vi "ORS_AlazarDLLCfg_All.vi"(2 "Bad Clock Duration":dbl=2.05e-06, 3 "Good Clock Duration":dbl=2.65e-06, 4 "DESmode":bool, 6 "IgnoreBadClk":bool, 7 "ATS_clock":T1={"Source"=2, "Sample Rate"=48, "Edge"=0, "Rate Ext Ref"=400000000, "Trigger Delay"=0, "Rate Int Ref"=450} {"Rate Ext Ref" items=["0.4G"=400000000, "0.8G"=800000000, "1.2G"=1200000000, "1.6G"=1600000000, "2.0G"=2000000000, "2.4G"=2400000000, "2.8G"=2800000000, "3.2G"=3200000000, "3.6G"=3600000000]; "Edge" items=["Rising", "Falling"]; "Sample Rate" items=["1 kS/s"=1, "2 kS/s"=2, "5 kS/s"=4, "10 kS/s"=8, "20 kS/s"=10, "50 kS/s"=12, "100 kS/s"=14, "200 kS/s"=16, "500 kS/s"=18, "1 MS/s"=20, "2 MS/s"=24, "5 MS/s"=26, "10 MS/s"=28, "20 MS/s"=30, "50 MS/s"=34, "100 MS/s"=36, "125 MS/s"=37, "200 MS/s"=40, "500 MS/s"=48, "800 MS/s"=50, "1000 MS/s"=53, "1200 MS/s"=55, "1500 MS/s"=58, "2000 MS/s"=63, "2400 MS/s"=106, "3000 MS/s"=117, "3600 MS/s"=123, "4000 MS/s"=128, "USER_DEF"=0]; "Source" items=["Internal"=1, "Fast External"=2, "Medium External"=3, "Slow External"=4, "External AC"=5, "External DC"=6, "External 10MHz"=7, "Internal 10MHz"=8]}, 8 "bufferCount":i32=128, 9 "Channel":u32(ring)=1 items=["A"=1, "B"=2, "A + B"=3, "C"=4, "A + C"=5, "A + B"=6, "D"=8, "A + D"=9, "B + D"=10, "C + D"=12, "A + B + C + D"=15], 10 "Range":u32(ring)=11 items=["20 mV"=1, "40 mV"=2, "50 mV"=3, "80 mV"=4, "100 mV"=5, "200 mV"=6, "400 mV"=7, "500 mV"=8, "800 mV"=9, "1 V"=10, "1.25 V"=33, "2 V"=11, "4 V"=12, "5 V"=13, "8 V"=14, "10 V"=15, "20 V"=16], 11 "System ID":u32=1) -> (0 "error out":errorcluster={"status"=FALSE, "code"=5512, "source"="OCT Ignore Bad Clock\rATS: ApiSuccess(512)"}, 5 "ATSHandle":u32=33760)   [LabVIEW 2024]
panel:
  out "Return Code":u32=512
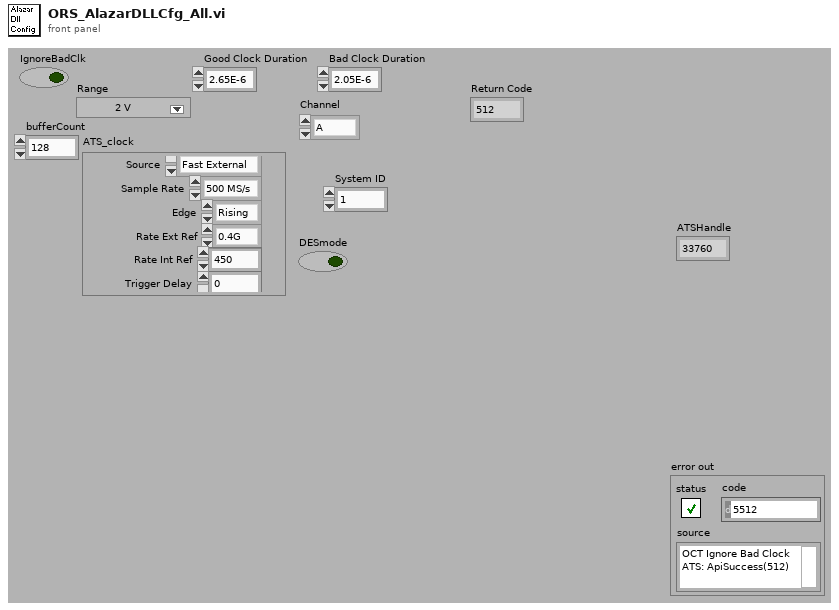
[diagram p1: front panel]
types:
  T1 = cluster{"Source":u32, "Sample Rate":u32, "Edge":u32, "Rate Ext Ref":u32, "Trigger Delay":u32, "Rate Int Ref":u32}
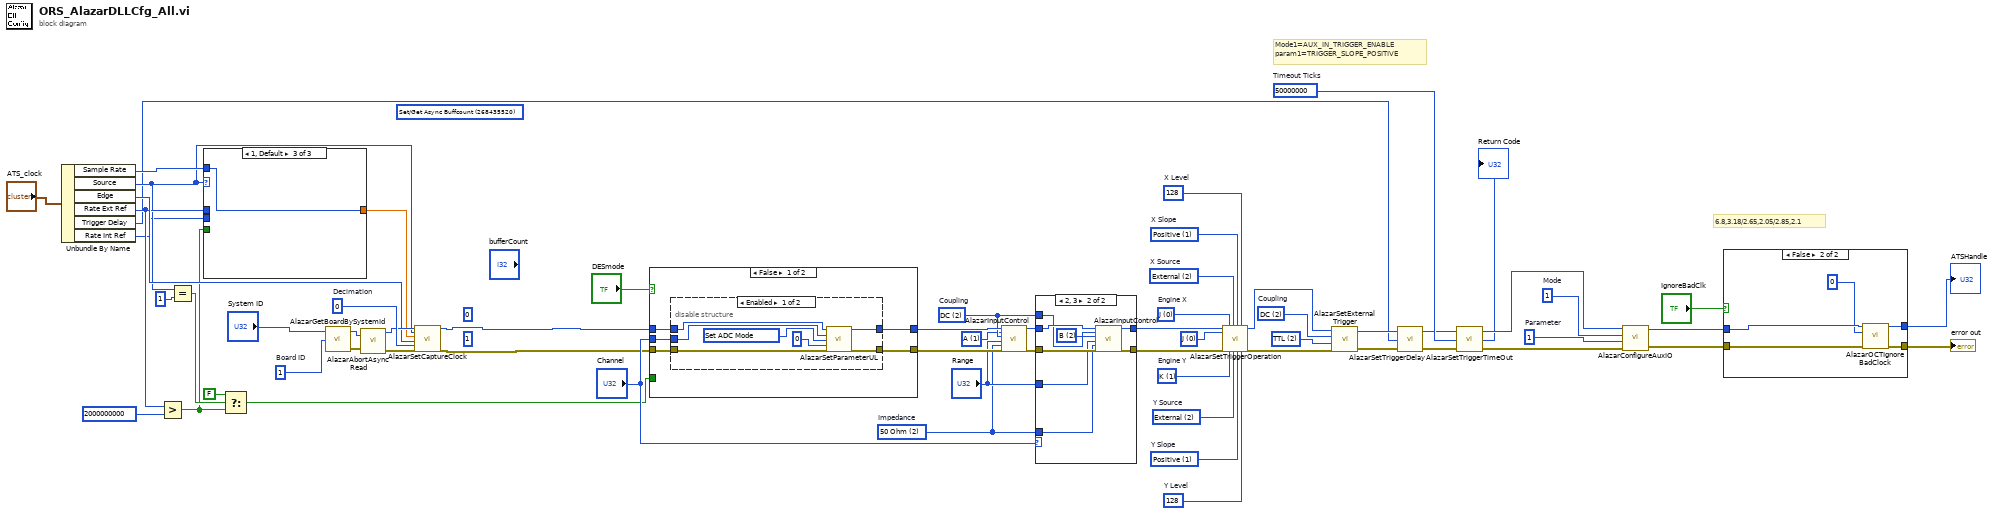
[diagram p0: block diagram]
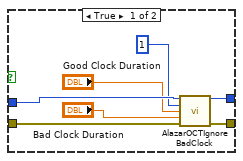
[diagram p2: hidden frame]
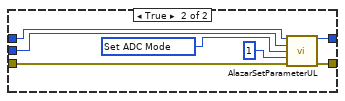
[diagram p5: hidden frame]
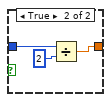
[diagram p7: hidden frame]
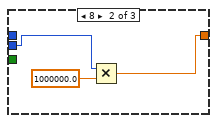
[diagram p8: hidden frame]
diagram:
  w5 = u32 1  # Parameter
  w6 = u32 1  # Mode
  w11 = u8 1 items=["A"=1, "B"=2, "C"=4, "D"=8] ("Channel")
  w21 = u32 2 items=["2.5V"=3, "5 V"=0, "1 V"=1, "TTL"=2] ("Range")
  (unwired) u32 268435520 items=["Set Single Chan."=268435523, "Data Width"=268435465, "Set/Get Async BuffSize"=268435513, "Set/Get Async Buffcount"=268435520, "Set Data Format"=268435521, "Get Data Format"=268435522, "Get Samples Per Timestamp Clock"=268435524, "Get Records Captured"=268435525, "Get Async Buffers Pending"=268435536, "Get Async Buffers Pending Full"=268435537, "Get Async Buffers Pending Empty"=268435538, "ECC Mode"=268435528, "Get Aux Input Level"=268435529, "Get Channels Per Board"=268435568, "Pack Mode"=268435570, "Get FPGA Temperature"=268435584] ("Parameter")
  (unwired) u8 0
  (unwired) 1 ("Value")
  w42 = u32 50000000  # Timeout Ticks
  w45 = u32 2 items=["AC"=1, "DC"=2]  # Coupling
  w54 = u32 128  # Y Level
  w53 = u32 1 items=["Positive"=1, "Negative"=2]  # Y Slope
  w52 = u32 2 items=["A", "B", "External", "Disable", "C", "D"]  # Y Source
  w50 = u32 128  # X Level
  w49 = u32 1 items=["Positive"=1, "Negative"=2]  # X Slope
  w48 = u32 2 items=["A", "B", "External", "Disable", "C", "D"]  # X Source
  w51 = u32 1 items=["J", "K"]  # Engine Y
  w47 = u32 0 items=["J", "K"]  # Engine X
  w46 = u32 0 items=["J", "K", "J OR K", "J AND K", "J XOR K", "J AND NOT K", "NOT J AND K"] ("Op.")
  w10 = u32 2 items=["50 Ohm"=2]  # Impedance
  w13 = u32 2 items=["DC"=2]  # Coupling
  w59 = u32 0  # Decimation
  w60 = u32 1  # Board ID
  # "6.8,3.18/2.65,2.05/2.85,2.1"
  # "Mode1=AUX_IN_TRIGGER_ENABLE\nparam1=TRIGGER_SLOPE_POSITIVE"
  n1 = Unbundle By Name("ATS_clock") -> ("Sample Rate"=w34:u32, "Source"=w28:u32, "Edge"=w33:u32, "Rate Ext Ref"=w32:u32, "Trigger Delay"=w23:u32, "Rate Int Ref"=w9:u32)
  n2 = Greater?(x=w32, y=u32 2000000000) -> (0:w25:bool)
  n3 = Equal?(x=w28, y=u32 1) -> (x = y?=w26:bool)
  n4 = case shown="1, Default" w28 {
    tunnel: w32 -> [w66 _ _]
    tunnel: w34 -> [_ _ w74]
    tunnel: w25 -> [w65 _ _]
    tunnel: w9 -> [_ w72 _]
    tunnel: [w64 w71 w74] -> w7
    frame 7 {
      n5 = case shown="False" w65 {
        tunnel: w66 -> [w67 w69]
        tunnel: [w67 w68] -> w64
        frame False {
        }
        frame True {
          n6 = Divide(x=w69, y=u32 2) -> (x/y=w68:dbl)
        }
      }
    }
    frame 8 {
      n7 = Multiply(x=w72, y=1000000.0) -> (x*y=w71:dbl)
    }
    frame 1, Default {
    }
  }
  n8 = Select(t=FALSE, s=w26, f=w25) -> (s? t:f=w3:bool)
  n9 = call "AlazarGetBoardBySystemId.vi"("Board ID"=w60, "System ID"="System ID") -> ("error out"=w56:errorcluster, "Handle"=w37:u32)  [unwired: 1 in, 1 out]
  n10 = call "AlazarAbortAsyncRead.vi"("Handle"=w37, "error in (no error)"=w56) -> ("Handle"=w58:u32, "error out"=w57:errorcluster)  [unwired: 1 out]
  n11 = call "AlazarSetCaptureClock.vi"("Handle"=w58, "Source"=w28, "Sample Rate"=w7, "Edge"=w33, "Decimation"=w59, "error in (no error)"=w57) -> ("Handle"=w2:u32, "error out"=w1:errorcluster)  [unwired: 11 in, 1 out]
  n12 = case shown="False" "DESmode" {
    tunnel: [w76 w95] -> w31
    tunnel: [w75 w94] -> w29
    tunnel: "Channel" -> [w78 w93]
    tunnel: w2 -> [w79 w92]
    tunnel: w1 -> [w77 w91]
    tunnel: w3 -> [_ _]
    frame False {
      n13 = disable-structure shown="Enabled" {
        disable-tunnel: w79 -> [w86 w88]
        disable-tunnel: w78 -> [w85 _]
        disable-tunnel: w77 -> [w84 w87]
        disable-tunnel: [w83 w87] -> w76
        disable-tunnel: [w82 w88] -> w75
        frame Enabled {
          w81 = u32 268435527 items=["Set ADC Mode"=268435527, "Data Width"=268435465, "Set/Get Async BuffSize"=268435513, "Set/Get Async Buffcount"=268435520, "Get Data Format"=268435522, "Get Samples Per Timestamp Clock"=268435524, "Get Records Captured"=268435525, "Get Async Buffers Pending"=268435536, "Get Async Buffers Pending Full"=268435537, "Get Async Buffers Pending Empty"=268435538, "ECC Mode"=268435528, "Get Aux Input Level"=268435529, "Get Channels Per Board"=268435568, "Pack Mode"=268435570, "Get FPGA Temperature"=268435584] ("Parameter")
          n14 = call "AlazarSetParameterUL.vi"("Handle"=w86, "Channel"=w85, "Parameter"=w81, "Value"=u32 0, "error in (no error)"=w84) -> ("Handle"=w82:u32, "error out"=w83:errorcluster)  [unwired: 8 in, 1 out]
        }
        frame Disabled {
        }
      }
    }
    frame True {
      w90 = u32 268435527 items=["Set ADC Mode"=268435527, "Data Width"=268435465, "Set/Get Async BuffSize"=268435513, "Set/Get Async Buffcount"=268435520, "Get Data Format"=268435522, "Get Samples Per Timestamp Clock"=268435524, "Get Records Captured"=268435525, "Get Async Buffers Pending"=268435536, "Get Async Buffers Pending Full"=268435537, "Get Async Buffers Pending Empty"=268435538, "ECC Mode"=268435528, "Get Aux Input Level"=268435529, "Get Channels Per Board"=268435568, "Pack Mode"=268435570, "Get FPGA Temperature"=268435584] ("Parameter")
      n15 = call "AlazarSetParameterUL.vi"("Handle"=w92, "Channel"=w93, "Parameter"=w90, "Value"=u32 1, "error in (no error)"=w91) -> ("Handle"=w94:u32, "error out"=w95:errorcluster)  [unwired: 8 in, 1 out]
    }
  }
  n16 = call "AlazarInputControl.vi"("Handle"=w29, "Channel"=w11, "Coupling"=w13, "Range"="Range", "Impedance"=w10, "error in (no error)"=w31) -> ("Handle"=w18:u32, "error out"=w16:errorcluster)  [unwired: 11 in, 1 out]
  n17 = case shown="2, 3" "Channel" {
    tunnel: w18 -> [w97 w105]
    tunnel: [w97 w104] -> w17
    tunnel: w16 -> [w96 w103]
    tunnel: [w96 w102] -> w15
    tunnel: "Range" -> [_ w101]
    tunnel: w13 -> [_ w100]
    tunnel: w10 -> [_ w98]
    frame 0, Default {
    }
    frame 2, 3 {
      w99 = u8 2 items=["A"=1, "B"=2, "C"=4, "D"=8] ("Channel")
      n18 = call "AlazarInputControl.vi"("Handle"=w105, "Channel"=w99, "Coupling"=w100, "Range"=w101, "Impedance"=w98, "error in (no error)"=w103) -> ("Handle"=w104:u32, "error out"=w102:errorcluster)  [unwired: 11 in, 1 out]
    }
  }
  n19 = call "AlazarSetTriggerOperation.vi"("Handle"=w17, "Operation"=w46, "error in (no error)"=w15, "Engine X"=w47, "Engine Y"=w51, "X Source"=w48, "Y Source"=w52, "X Slope"=w49, "Y Slope"=w53, "X Level"=w50, "Y Level"=w54) -> ("Handle"=w44:u32, "error out"=w43:errorcluster)  [unwired: 6 in, 1 out]
  n20 = call "AlazarSetExternalTrigger.vi"("error in (no error)"=w43, "Range"=w21, "Coupling"=w45, "Handle"=w44) -> ("error out"=w38:errorcluster, "Handle"=w39:u32)  [unwired: 1 out]
  n21 = call "AlazarSetTriggerDelay.vi"("error in (no error)"=w38, "Value"=w23, "Handle"=w39) -> ("error out"=w41:errorcluster, "Handle"=w40:u32)  [unwired: 1 out]
  n22 = call "AlazarSetTriggerTimeOut.vi"("error in (no error)"=w41, "Timeout Ticks"=w42, "Handle"=w40) -> ("error out"=w35:errorcluster, "Return Code"=→"Return Code":u32, "Handle"=w36:u32)
  n23 = call "AlazarConfigureAuxIO.vi"("error in (no error)"=w35, "Parameter"=w5, "Mode"=w6, "Handle"=w36) -> ("error out"=w19:errorcluster, "Handle"=w20:u32)  [unwired: 1 out]
  n24 = case shown="False" "IgnoreBadClk" {
    tunnel: [w112 w117] -> w63
    tunnel: [w111 w116] -> w62
    tunnel: w20 -> [w110 w115]
    tunnel: w19 -> [w109 w114]
    frame True {
      n25 = call "AlazarOCTIgnoreBadClock.vi"("Handle"=w110, "Enable"=u32 1, "Good Clock Duration"="Good Clock Duration", "Bad Clock Duration"="Bad Clock Duration", "error in (no error)"=w109) -> ("Handle"=w111:u32, "error out"=w112:errorcluster)  [unwired: 6 in, 3 out]
    }
    frame False {
      n26 = call "AlazarOCTIgnoreBadClock.vi"("Handle"=w115, "Enable"=u32 0, "error in (no error)"=w114) -> ("Handle"=w116:u32, "error out"=w117:errorcluster)  [unwired: 8 in, 3 out]
    }
  }
  "error out" <- w63
  "ATSHandle" <- w62
